vi "RWA-Test.vi"() -> ()   [LabVIEW 2015]
panel:
  in  "FuckYou":dbl
  out "Indicator":string
  in  "Cluster":T1
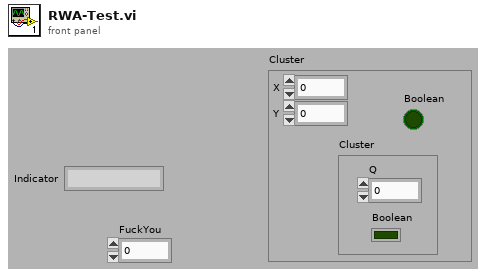
[diagram p1: front panel]
types:
  T1 = cluster{"X":dbl, "Y":dbl, "Cluster":cluster{"Q":dbl, "Boolean":bool}, "Boolean":bool}
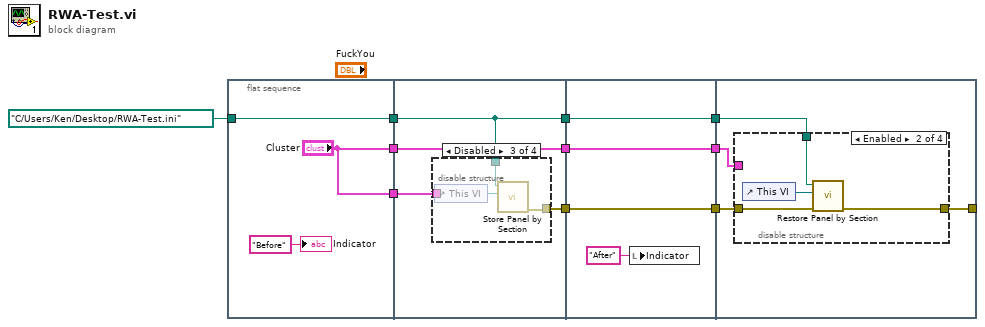
[diagram p0: block diagram]
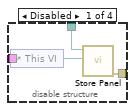
[diagram p2: hidden frame]
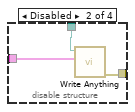
[diagram p3: hidden frame]
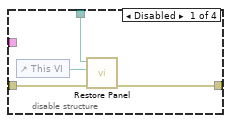
[diagram p5: hidden frame]
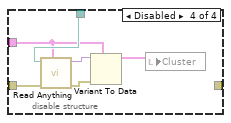
[diagram p7: hidden frame]
diagram:
  n1 = flat-sequence {
    tunnel: [w12] -> w10
    tunnel: path "C:/Users/Ken/Desktop/RWA-Test.ini" ("Path (dialog)") -> [w12]
    tunnel: ["Cluster"] -> w4
    tunnel: ["Cluster"] -> w1
    tunnel: w10 -> [w14]
    tunnel: [w17] -> w8
    tunnel: [w14] -> w5
    tunnel: w4 -> [w15]
    tunnel: [w16] -> w2
    tunnel: w1 -> [w16]
    tunnel: w8 -> [w30]
    tunnel: [w30] -> w7
    tunnel: [w28] -> w6
    tunnel: w5 -> [w28]
    tunnel: [w27] -> w3
    tunnel: w2 -> [w27]
    tunnel: [w33] -> _
    tunnel: w7 -> [w34]
    tunnel: w6 -> [w32]
    tunnel: w3 -> [w31]
    frame #0 {
      "Indicator" <- "Before" ("Indicator")
    }
    frame #1 {
      n2 = disable-structure shown="Disabled" {
        disable-tunnel: [w19 w23 w26 _] -> w17
        disable-tunnel: w15 -> [_ w21 _ _]
        disable-tunnel: w14 -> [w18 w22 w25 _]
        frame Disabled {
          n3 = control-ref of="This VI"() -> (w20:refnum<vi>)
          n4 = call "Store Panel.vi"("VI reference"=w20, "Path (dialog)"=w18) -> ("Error Out"=w19:errorcluster)  [unwired: 9 in]
        }
        frame Disabled {
          n5 = call "Write Anything.vi"("Anything"=w21, "Path (dialog)"=w22) -> ("Error Out"=w23:errorcluster)  [unwired: 8 in, 1 out]
        }
        frame Disabled {
          n6 = control-ref of="This VI"() -> (w24:refnum<vi>)
          n7 = call "Store Panel by Section.vi"("VI reference"=w24, "Path (dialog)"=w25) -> ("Error Out"=w26:errorcluster)  [unwired: 9 in]
        }
        frame Enabled {
        }
      }
    }
    frame #2 {
      n8 = local write "Indicator"("After" ("Indicator")) -> ()
    }
    frame #3 {
      n9 = disable-structure shown="Enabled" {
        disable-tunnel: w34 -> [w38 w42 _ w48]
        disable-tunnel: [w37 w41 _ _] -> w33
        disable-tunnel: w32 -> [w36 w40 _ w47]
        disable-tunnel: w31 -> [_ _ _ w44]
        frame Disabled {
          n10 = control-ref of="This VI"() -> (w35:refnum<vi>)
          n11 = call "Restore Panel.vi"("Error In"=w38, "VI reference"=w35, "Path (dialog)"=w36) -> ("error out"=w37:errorcluster)  [unwired: 8 in]
        }
        frame Enabled {
          n12 = control-ref of="This VI"() -> (w39:refnum<vi>)
          n13 = call "Restore Panel by Section.vi"("error in (no error)"=w42, "VI reference"=w39, "Path (dialog)"=w40) -> ("Error Out"=w41:errorcluster)  [unwired: 8 in]
        }
        frame Disabled {
        }
        frame Disabled {
          n14 = call "Read Anything.vi"("Type of Anything"=w44, "Error In"=w48, "Path (dialog)"=w47) -> ("Error Out"=w46:errorcluster, "Anything"=w45:variant)  [unwired: 6 in, 1 out]
          n15 = Variant To Data(error in=w46, type=w44, Variant=w45) -> (data=w43:T1)  [unwired: 1 out]
          n16 = local write "Cluster"(w43) -> ()
        }
      }
    }
  }
